vi "ms.vi"(1 "Reset":bool) -> (0 "millisecond":u32)   [LabVIEW 2016]
doc: "This VI uses the elapsed Miliseconds VI for timing but upon intialization it zeros the current time. This avoids timing complications caused by the function not always starting at zero. It also allows the user to restart the time by sending true to the reset terminal.\n\nCreated by Team 4130 for use in the 2016-2017 FRC season"
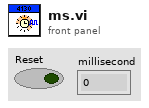
[diagram p1: front panel]
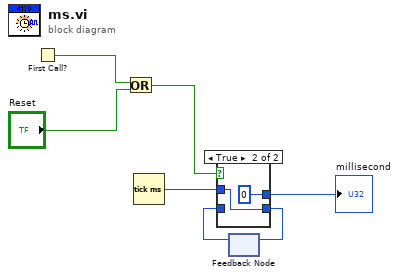
[diagram p0: block diagram]
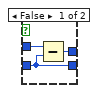
[diagram p2: hidden frame]
diagram:
  n1 = First Call?() -> (First Call?: T/F=w3:bool)
  n2 = Or(x=w3, y="Reset") -> (x .or. y?=w2:bool)
  n3 = Tick Count (ms)() -> (millisecond timer value=w4:u32)
  n4 = feedback #1() -> (w6:u32)  [unwired: 1 in]
  n5 = case shown="True" w2 {
    tunnel: w4 -> [w10 w12]
    tunnel: [w9 u32 0] -> w7
    tunnel: [w8 w12] -> w5
    tunnel: w6 -> [w8 _]
    frame False {
      n6 = Subtract(x=w10, y=w8) -> (x-y=w9:u32)
    }
    frame True {
    }
  }
  "millisecond" <- w7
  n7 = feedback-in #1(w5) -> ()
